vi "FIR Filtering Using Optional Specs.vi"() -> ()   [LabVIEW 2023]
doc: "Demonstrates the use of the optional filter specifications cluster, allowing an alternate method of specifying Equi-ripple FIR filters."
uses:
  <vilib>/measure/macond.llb/FIR Filter for 1 Chan.vi
  <vilib>/measure/NI_MABase.lvlib
  <vilib>/measure/NI_MAPro.lvlib
panel:
  in  "Tab Control":T1(tab)
  out "Waveform Graph":waveform(dbl)[](graph)
  out "Magnitude response":cluster{"f0":dbl, "df":dbl, "Mag H(w)":dbl[]}(graph)={"f0"=0.0, "df"=0.9765625, "Mag H(w)"=[]}
  out "Phase response":cluster{"f0":dbl, "df":dbl, "Phase H(w)":dbl[]}(graph)={"f0"=0.0, "df"=0.9765625, "Phase H(w)"=[]}
  out "order":i32
  in  "noise amplitude":dbl(slide)=0.9591836734693877 scale=0.0..2.0
  in  "optional FIR filter specifications":T2={"PB Gain"=0.01, "SB Gain"=-60.0, "Scale"=TRUE, "Window"=enum."None"} {"SB Gain" format="%#.6g"; "PB Gain" format="%#.6g"}
  in  "reset signal":bool
  in  "FIR filter specifications":T3={"Topology"=enum."FIR by Specification", "Type"=enum."Lowpass", "# Taps"=32, "Lower PB"=100.0, "Upper PB"=0.0, "Lower SB"=200.0, "Upper SB"=0.0} {"Upper SB" format="%#.6g"; "Lower SB" format="%#.6g"; "Upper PB" format="%#.6g"; "Lower PB" format="%#.6g"}
  in  "reset filter":bool
  in  "sampling info":cluster{"Fs":dbl, "#s":dbl}={"Fs"=1000.0, "#s"=100.0} {"#s" step=100.0 format="%#.6g"; "Fs" step=1000.0 format="%#.6g"}
  in  "signal parameters":T4={"signal type"=enum."Square Wave", "frequency"=100.0} {"frequency" format="%#.6g"}
  in  "Stop":bool
  # "Overview: Demonstrates the use of the \"optional FIR filter specification\" input to the Digital FIR Filter VI.\nRequirements: LabVIEW Full Development System\nInstructions: \n1. Run the VI. \n2. Notice that the # Taps and Window controls are disabled.\n3. Select the Filter Information tab.\n4. Change the optional FIR filter specification values and notice the effect on the order value.\n5. Click Stop to stop the VI."
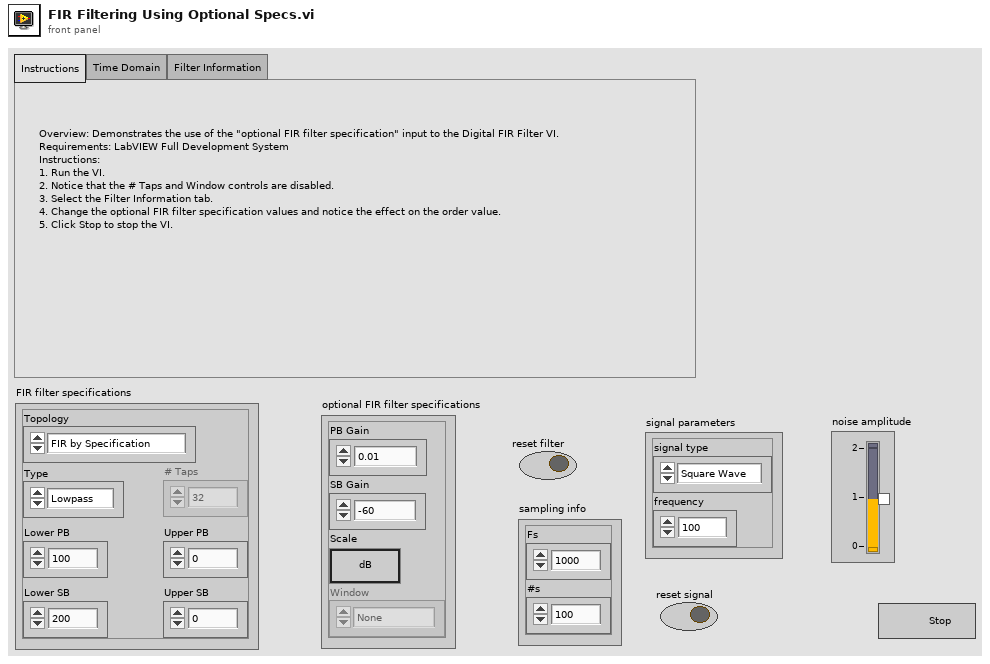
[diagram p1: front panel]
types:
  T1 = enum32{"Instructions", "Time Domain", "Filter Information"}
  T2 = cluster{"PB Gain":dbl, "SB Gain":dbl, "Scale":bool, "Window":enum16{"None", "Hanning", "Hamming", "Triangular", "Blackman", "Exact Blackman", "Blackman-Harris", "Kaiser-Bessel", "Flat Top"}}
  T3 = cluster{"Topology":enum16{"Off", "FIR by Specification", "Equi-ripple FIR", "Windowed FIR"}, "Type":enum16{"Lowpass", "Highpass", "Bandpass", "Bandstop"}, "# Taps":i32, "Lower PB":dbl, "Upper PB":dbl, "Lower SB":dbl, "Upper SB":dbl}
  T4 = cluster{"signal type":enum16{"Sine Wave", "Triangle Wave", "Square Wave", "Sawtooth Wave"}, "frequency":dbl}
  T5 = enum16{"Sine Wave", "Triangle Wave", "Square Wave", "Sawtooth Wave"}
  T6 = cluster{"magnitude H(w)":cluster{"f0":dbl, "df":dbl, "Mag H(w)":dbl[]}, "phase H(w)":cluster{"f0":dbl, "df":dbl, "Phase H(w)":dbl[]}, "order":i32}
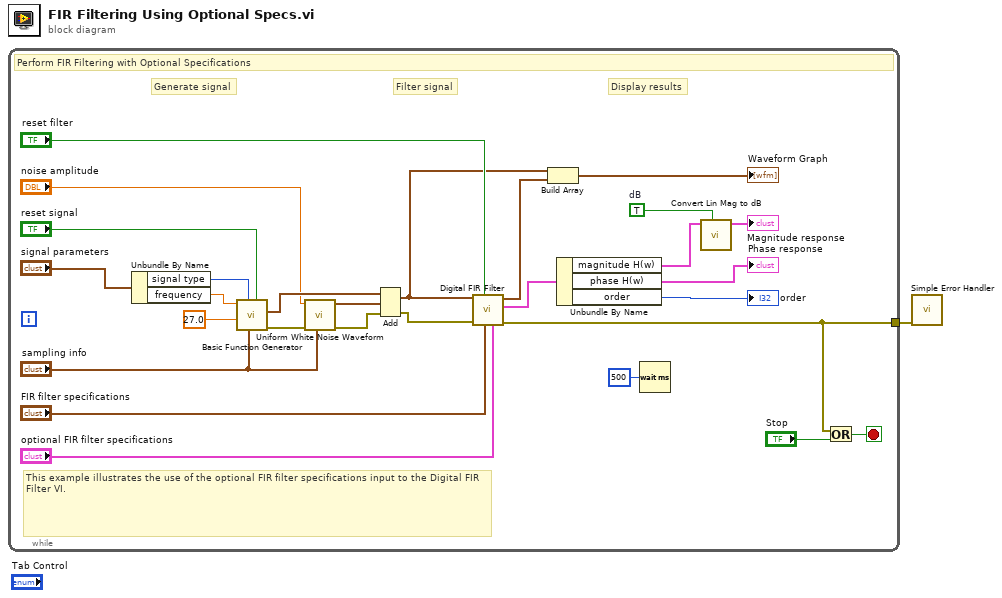
[diagram p0: block diagram]
diagram:
  n1 = while {
    tunnel: [w3] -> w1
    stop <- w13 stop-if-true
    w5 = TRUE  # dB
    # "This example illustrates the use of the optional FIR filter specifications input to the Digital FIR Filter VI."
    # "Display results"
    # "Filter signal"
    # "Generate signal"
    # "Perform FIR Filtering with Optional Specifications"
    n2 = Unbundle By Name("signal parameters") -> ("signal type"=w25:T5, "frequency"=w2:dbl)
    n3 = call <vilib>:"Basic Function Generator.vi"("reset signal"="reset signal", "sampling info"="sampling info", "signal type"=w25, "phase"=27.0, "frequency"=w2) -> ("error out"=w20:errorcluster, "signal out"=w16:waveform(dbl))  [unwired: 4 in, 1 out]
    n4 = call <vilib>:"Uniform White Noise Waveform.vi"("sampling info"="sampling info", "error in (no error)"=w20, "amplitude"="noise amplitude") -> ("error out"=w19:errorcluster, "signal out"=w17:waveform(dbl))  [unwired: 7 in]
    n5 = Add(1:w17, 2:w16, 4:w19) -> (0:w11:waveform(dbl), 3:w18:errorcluster)
    n6 = call-poly <vilib>:"Digital FIR Filter.vi"("optional FIR filter specifications"="optional FIR filter specifications", "FIR filter specifications"="FIR filter specifications", "reset filter"="reset filter", "error in (no error)"=w18, "signal in"=w11) -> ("error out"=w3:errorcluster, "filter information"=w14:T6, "signal out"=w10:waveform(dbl))  [unwired: 4 in]
    n7 = Build Array(w11, w10) -> (→"Waveform Graph":waveform(dbl)[])
    n8 = Unbundle By Name(w14) -> ("magnitude H(w)"=w9:cluster{"f0":dbl, "df":dbl, "Mag H(w)":dbl[]}, "phase H(w)"=→"Phase response":cluster{"f0":dbl, "df":dbl, "Phase H(w)":dbl[]}, "order"=→"order":i32)
    n9 = Wait (ms)(milliseconds to wait=u32 500) -> ()  [unwired: 1 out]
    n10 = call "Convert Lin Mag to dB.vi"("convert to dB"=w5, "magnitude H(w)"=w9) -> ("magnitude H(w) in dB"=→"Magnitude response":cluster{"f0":dbl, "df":dbl, "Mag H(w)":dbl[]})  [unwired: 9 in]
    n11 = Or(x=w3, y="Stop") -> (x .or. y?=w13:bool)
  }
  n12 = call <vilib>:"Simple Error Handler.vi"("error in (no error)"=w1) -> ()  [unwired: 4 in, 5 out]
